vi "LUNCHER.vi"   [LabVIEW 2023]
uses:
  Labview/img_data.ctl
  <vilib>/picture/picture.llb/imagedata.ctl
  Labview/data_commands.ctl
  tcp_enum.ctl
  Labview/data.ctl
  Labview/commands.ctl
types:
  T1 = typedef "data.ctl" = cluster{"gui_commands":T2, "curent":T3, "ori":T3}
  T2 = typedef "commands.ctl" = enum16{"display", "bin", "gauss", "edg", "blurr", "connect", "stop", "idle"}
  T3 = typedef "imagedata.ctl" = cluster{"image type":i32, "image depth":i32, "image":u8[], "mask":u8[], "colors":u32[], "Rectangle":cluster{"left":i16, "top":i16, "right":i16, "bottom":i16}}
  T4 = typedef "img_data.ctl" = cluster{"ori":T3, "curent":T3, "comands":T5}
  T5 = typedef "data_commands.ctl" = enum16{"stop", "bin", "edg", "gauss", "blurr", "idle"}
  T6 = typedef "tcp_enum.ctl" = enum16{"idle", "stop", "connect"}
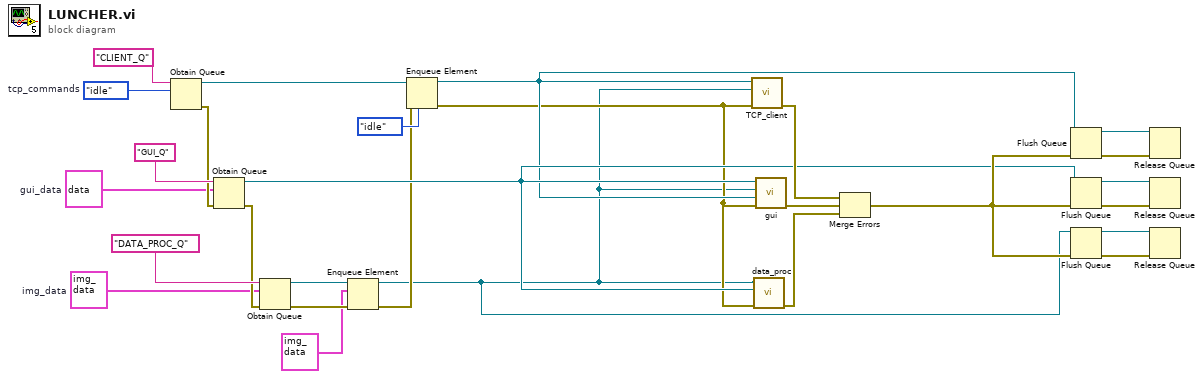
[diagram p0: block diagram]
diagram:
  w1 = T1 {"gui_commands"=enum."bin", "curent"={"image type"=0, "image depth"=0, "image"=[], "mask"=[], "colors"=[], "Rectangle"={"left"=0, "top"=0, "right"=0, "bottom"=0}}, "ori"={"image type"=0, "image depth"=0, "image"=[], "mask"=[], "colors"=[], "Rectangle"={"left"=0, "top"=0, "right"=0, "bottom"=0}}}  # gui_data
  w19 = T4 {"ori"={"image type"=0, "image depth"=0, "image"=[], "mask"=[], "colors"=[], "Rectangle"={"left"=0, "top"=0, "right"=0, "bottom"=0}}, "curent"={"image type"=0, "image depth"=0, "image"=[], "mask"=[], "colors"=[], "Rectangle"={"left"=0, "top"=0, "right"=0, "bottom"=0}}, "comands"=enum."stop"}  # img_data
  w20 = tcp_enum."idle"  # tcp_commands
  n1 = Obtain Queue(name (unnamed)="CLIENT_Q", element data type=w20) -> (queue out=w10:refnum<queue>, error out=w25:errorcluster)  [unwired: 3 in, 1 out]
  n2 = Obtain Queue(name (unnamed)="GUI_Q", element data type=w1, error in (no error)=w25) -> (queue out=w11:refnum<queue>, error out=w24:errorcluster)  [unwired: 2 in, 1 out]
  n3 = Obtain Queue(name (unnamed)="DATA_PROC_Q", element data type=w19, error in (no error)=w24) -> (queue out=w7:refnum<queue>, error out=w5:errorcluster)  [unwired: 2 in, 1 out]
  n4 = Enqueue Element(queue=w7, element=T4 {"ori"={"image type"=0, "image depth"=0, "image"=[], "mask"=[], "colors"=[], "Rectangle"={"left"=0, "top"=0, "right"=0, "bottom"=0}}, "curent"={"image type"=0, "image depth"=0, "image"=[], "mask"=[], "colors"=[], "Rectangle"={"left"=0, "top"=0, "right"=0, "bottom"=0}}, "comands"=enum."idle"} ("img_data"), error in (no error)=w5) -> (queue out=w3:refnum<queue>, error out=w4:errorcluster)  [unwired: 1 in, 1 out]
  n5 = Enqueue Element(queue=w10, element=tcp_enum."idle" ("tcp_commands"), error in (no error)=w4) -> (queue out=w9:refnum<queue>, error out=w6:errorcluster)  [unwired: 1 in, 1 out]
  n6 = call "TCP_client.vi"("error in (no error)"=w6, "data_q"=w3, "client"=w9) -> ("error out"=w21:errorcluster)  [unwired: 8 in]
  n7 = call "data_proc.vi"("error out 2"=w6, "gui_q"=w11, "data_q"=w3) -> ("error out"=w22:errorcluster)  [unwired: 8 in]
  n8 = call "gui.vi"("error in (no error)"=w6, "client_q"=w9, "data_q"=w3, "gui_q"=w11) -> ("error out"=w23:errorcluster)  [unwired: 7 in]
  n9 = Merge Errors(w21, w23, w22) -> (w18:errorcluster)
  n10 = Flush Queue(queue=w9, error in (no error)=w18) -> (queue out=w14:refnum<queue>, error out=w17:errorcluster)  [unwired: 1 out]
  n11 = Flush Queue(queue=w11, error in (no error)=w18) -> (queue out=w13:refnum<queue>, error out=w16:errorcluster)  [unwired: 1 out]
  n12 = Flush Queue(queue=w3, error in (no error)=w18) -> (queue out=w12:refnum<queue>, error out=w15:errorcluster)  [unwired: 1 out]
  n13 = Release Queue(queue=w14, error in (no error)=w17) -> ()  [unwired: 1 in, 3 out]
  n14 = Release Queue(queue=w13, error in (no error)=w16) -> ()  [unwired: 1 in, 3 out]
  n15 = Release Queue(queue=w12, error in (no error)=w15) -> ()  [unwired: 1 in, 3 out]
